vi "Read Multicolumn Listbox Headers (UTF-8 String).vi"(8 "error in":errorcluster, 11 "Control Ref":refnum<vi>) -> (0 "error out":errorcluster, 1 "Row Headers":refnum<class "UTF-8 String.lvclass">[](array[class]), 2 "Column Headers":refnum<class "UTF-8 String.lvclass">[](array[class]))   [LabVIEW 2020, in "G-Unicode.lvlib"]
doc: "Read unicode text from a control or text element of a control. If the control text is not unicode, it will be converted to unicode."
uses:
  G-Unicode.lvlib
  f6f7f231-7ddf-476b-a943-0386d848a5c9.vi
  fba5a6d2-cdfe-4afc-9e2c-d2641906be0d.vi
  Types/UTF-8 String/UTF-8 String.lvclass
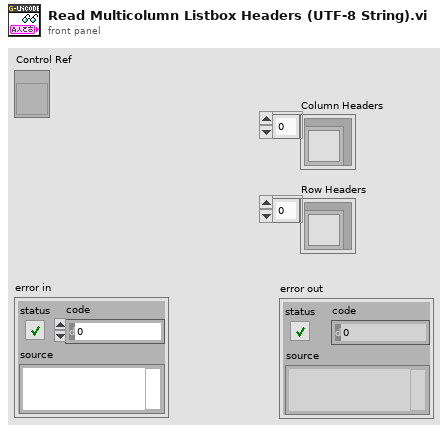
[diagram p1: front panel]
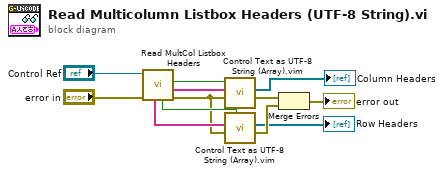
[diagram p0: block diagram]
diagram:
  n1 = call "Read MultCol Listbox Headers.vi"("error in"="error in", "Multicolumn Listbox Ref in"="Control Ref") -> ("error out"=w5:errorcluster, "Column Headers"=w10:string[], "Interpret As Unicode (Columns)"=w9:bool, "Interpret As Unicode (Rows)"=w7:bool, "Row Headers"=w6:string[])  [unwired: 4 in, 1 out]
  n2 = call "Control Text as UTF-8 String (Array).vim"("Interpret As Unicode"=w9, "error in"=w5, "Control Text"=w10) -> ("error out"=w4:errorcluster, "UTF-8 String"=→"Column Headers":refnum<class "UTF-8 String.lvclass">[])  [unwired: 7 in]
  n3 = call "Control Text as UTF-8 String (Array).vim"("Interpret As Unicode"=w7, "error in"=w5, "Control Text"=w6) -> ("error out"=w3:errorcluster, "UTF-8 String"=→"Row Headers":refnum<class "UTF-8 String.lvclass">[])  [unwired: 7 in]
  n4 = Merge Errors(w4, w3) -> (→"error out":errorcluster)
